vi "CTRE_Phoenix_CANcoder_ConfigAllSettings.vi"(6 "timeoutMs":i32=50, 7 "Force Write":bool, 8 "error in (no error)":errorcluster, 10 "CANcoder Configurables":T1={"Sensor Initialization Strategy"=enum."Boot To Zero", "Absolute Sensor Range"=enum."Unsigned [0 to 360)", "Velocity Measurement Period"=100, "Velocity Measurement Window"=64, "Magnet Offset (Degrees)"=0.0, "Sensor Direction"=FALSE, "Sensor Coefficient"=0.087890625, "Unit String"="deg", "Sensor Time Base"=enum."PerMinute"} {"Velocity Measurement Period" items=["Period_1ms"=1, "Period_2ms"=2, "Period_5ms"=5, "Period_10ms"=10, "Period_20ms"=20, "Period_25ms"=25, "Period_50ms"=50, "Period_100ms"=100]; "Sensor Coefficient" format="%#_9g"}, 11 "CTRE_CANcoder_DeviceRef":T6) -> (0 "error out":errorcluster, 3 "CTRE_CANcoder_DeviceRef":T6)   [LabVIEW 2019]
doc: "Configures all persistent settings of the CANcoder.\n\n<b>CANcoder Configurables</b> Cluster of configurable settings. Using a \"control\" on the calling VI's front panel will display documentation for each setting."
uses:
  <vilib>/Rock Robotics/WPI/ThirdParty/Phoenix-LabVIEW/CANCoder/Controls/CTRE_Phoenix_CANcoder_DeviceRef.ctl
  <vilib>/Rock Robotics/WPI/ThirdParty/Phoenix-LabVIEW/CANCoder/Controls/CTRE_Phoenix_CANcoder_Configurables.ctl
  <vilib>/Rock Robotics/WPI/ThirdParty/Phoenix-LabVIEW/CANCoder/Controls/CTRE_Phoenix_CANcoder_SensorInitializationStrategy.ctl
  <vilib>/Rock Robotics/WPI/ThirdParty/Phoenix-LabVIEW/CANCoder/Controls/CTRE_Phoenix_CANcoder_AbsoluteSensorRange.ctl
  <vilib>/Rock Robotics/WPI/ThirdParty/Phoenix-LabVIEW/Motor Controller/Controls/CTRE_Phoenix_MotorControl_VelocityMeasurementPeriod.ctl
  <vilib>/Rock Robotics/WPI/ThirdParty/Phoenix-LabVIEW/CANCoder/Controls/CTRE_Phoenix_CANcoder_SensorTimeBase.ctl
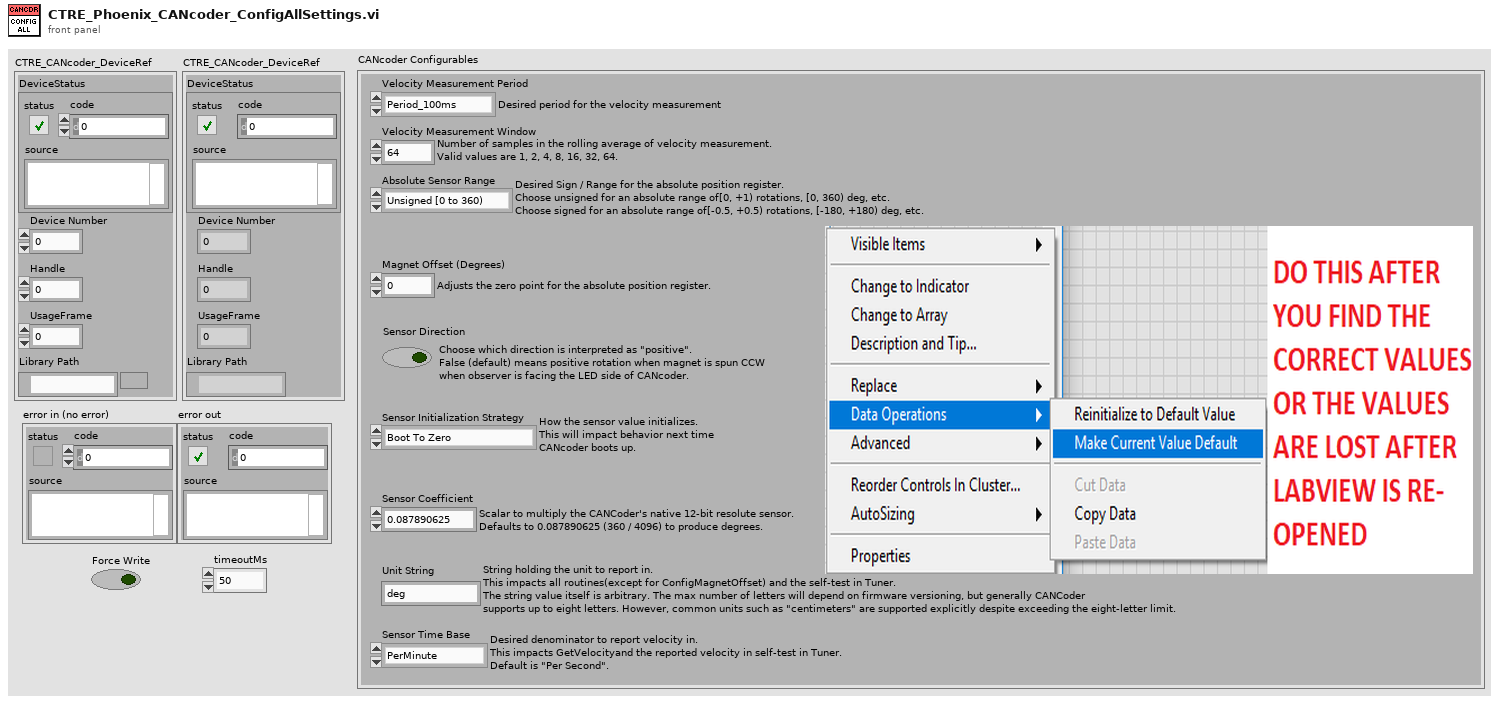
[diagram p1: front panel]
types:
  T1 = typedef "CTRE_Phoenix_CANcoder_Configurables.ctl" = cluster{"Sensor Initialization Strategy":T2, "Absolute Sensor Range":T3, "Velocity Measurement Period":T4, "Velocity Measurement Window":i32, "Magnet Offset (Degrees)":dbl, "Sensor Direction":bool, "Sensor Coefficient":dbl, "Unit String":string, "Sensor Time Base":T5}
  T2 = typedef "CTRE_Phoenix_CANcoder_SensorInitializationStrategy.ctl" = enum16{"Boot To Zero", "Boot To Absolute Position"}
  T3 = typedef "CTRE_Phoenix_CANcoder_AbsoluteSensorRange.ctl" = enum16{"Unsigned [0 to 360)", "Signed [-180 to +180)"}
  T4 = typedef "CTRE_Phoenix_MotorControl_VelocityMeasurementPeriod.ctl" = u16
  T5 = typedef "CTRE_Phoenix_CANcoder_SensorTimeBase.ctl" = enum16{"Per100Ms_Legacy", "PerSecond", "PerMinute"}
  T6 = typedef "CTRE_Phoenix_CANcoder_DeviceRef.ctl" = cluster{"DeviceStatus":errorcluster, "Device Number":u8, "Handle":u64, "UsageFrame":u32, "Library Path":path}
  T7 = cluster{"Sensor Initialization Strategy":bool, "Absolute Sensor Range":bool, "Velocity Measurement Period":bool, "Velocity Measurement Window":bool, "Magnet Offset (Degrees)":bool, "Sensor Direction":bool, "Sensor Coefficient":bool, "Unit String":bool, "Sensor Time Base":bool}
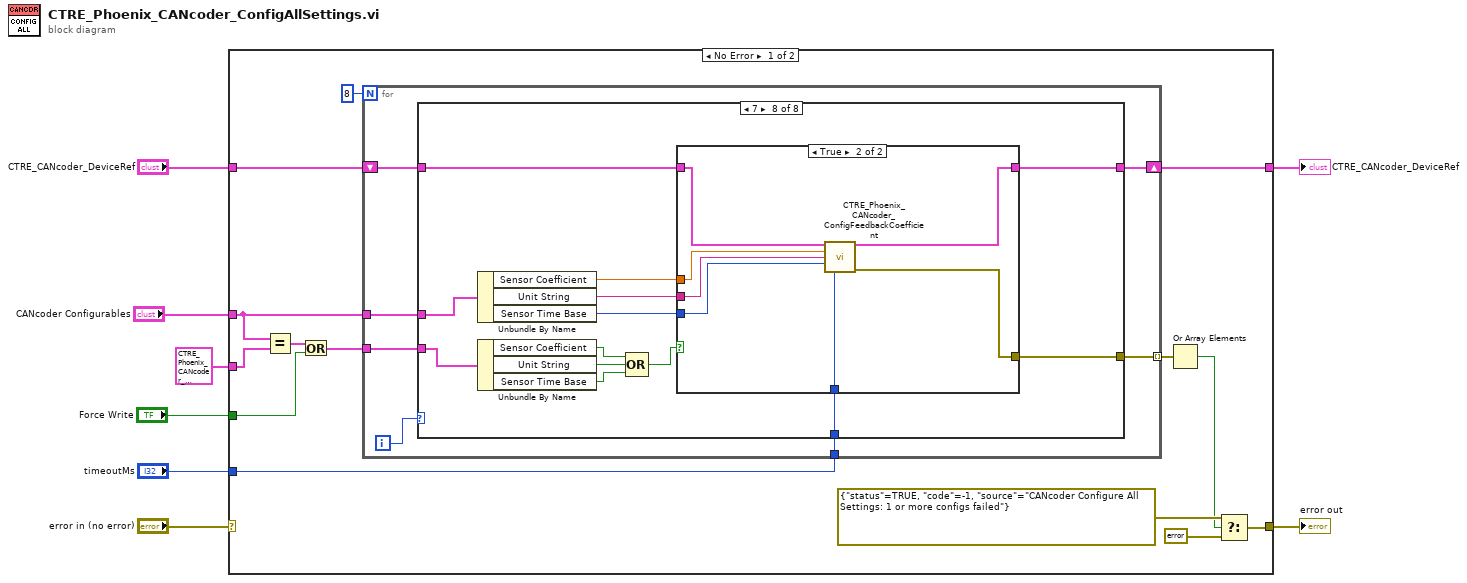
[diagram p0: block diagram]
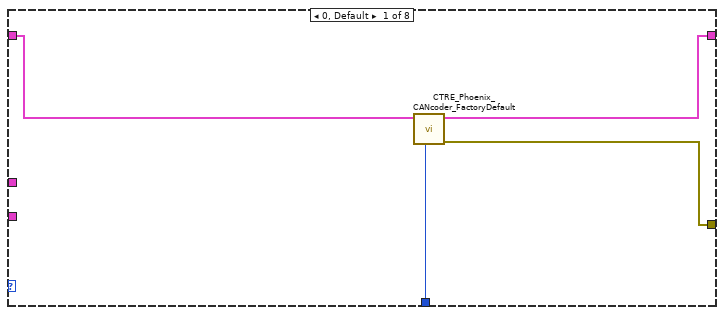
[diagram p2: hidden frame]
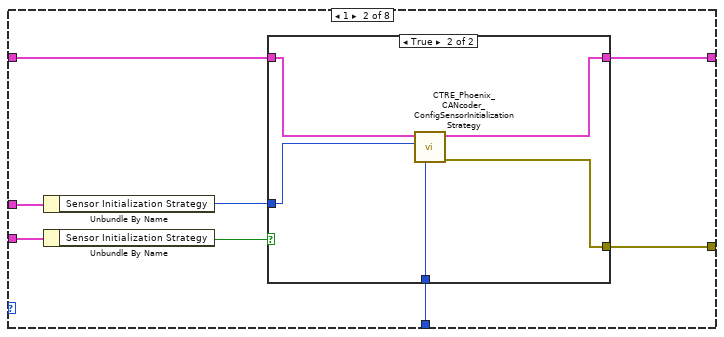
[diagram p3: hidden frame]
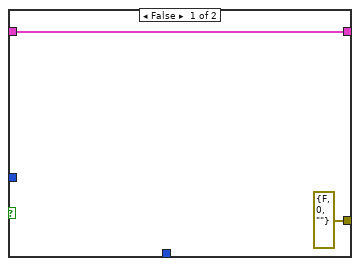
[diagram p4: hidden frame]
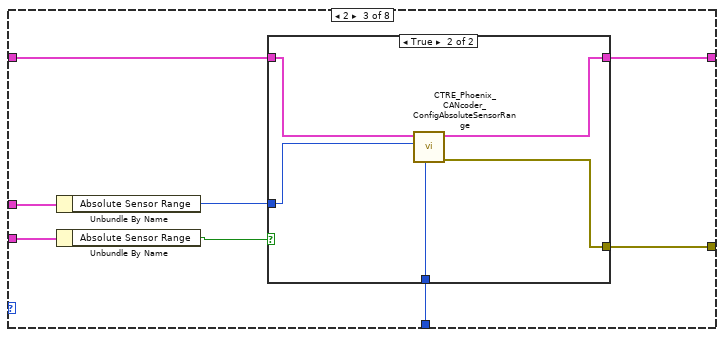
[diagram p5: hidden frame]
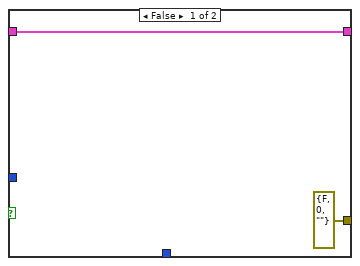
[diagram p6: hidden frame]
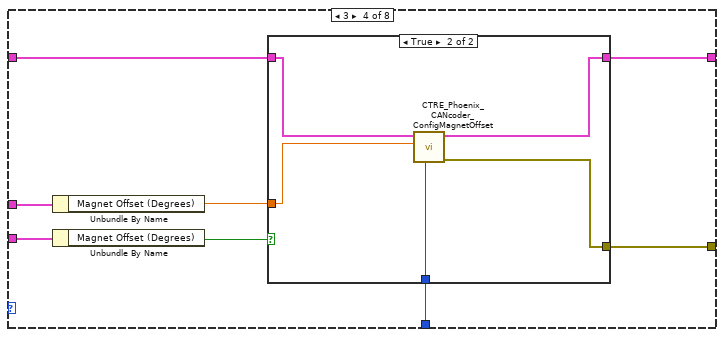
[diagram p7: hidden frame]
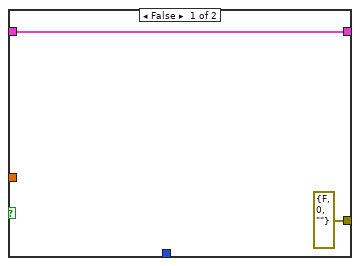
[diagram p8: hidden frame]
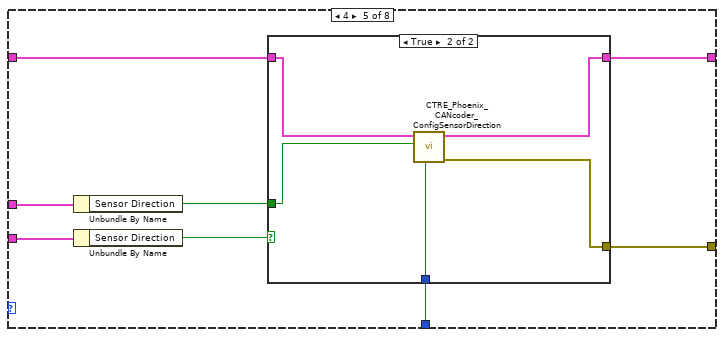
[diagram p9: hidden frame]
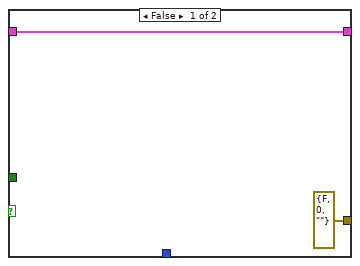
[diagram p10: hidden frame]
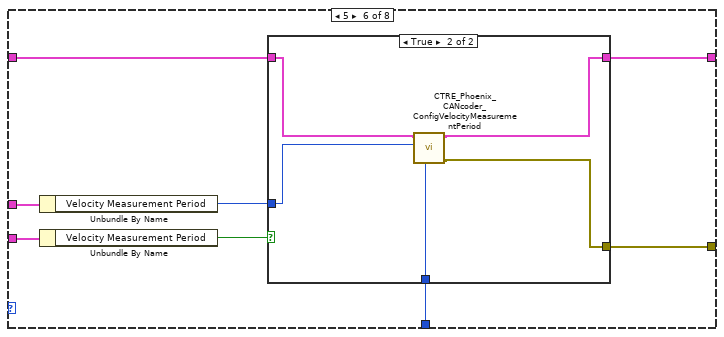
[diagram p11: hidden frame]
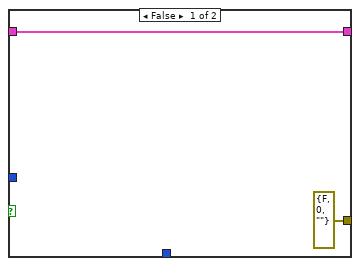
[diagram p12: hidden frame]
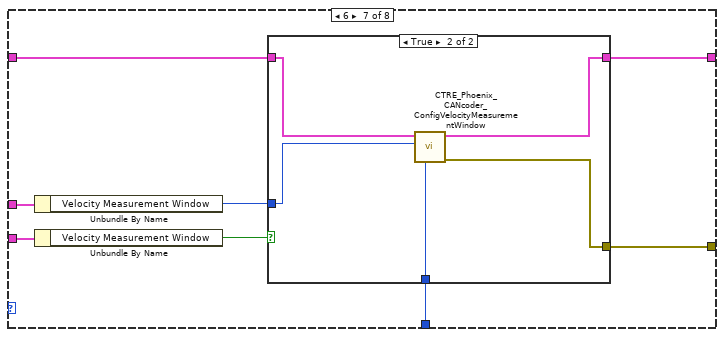
[diagram p13: hidden frame]
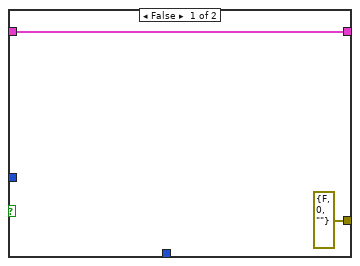
[diagram p14: hidden frame]
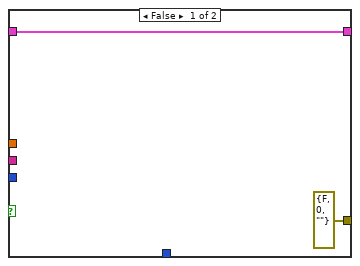
[diagram p15: hidden frame]
diagram:
  n1 = case shown="No Error" "error in (no error)" {
    selector: "error in (no error)" -> [_ w146]
    tunnel: "CTRE_CANcoder_DeviceRef" -> [w19 w147]
    tunnel: [w9 w147] -> w6
    tunnel: [w11 w146] -> w5
    tunnel: "timeoutMs" -> [w15 _]
    tunnel: "Force Write" -> [w20 _]
    tunnel: "CANcoder Configurables" -> [w16 _]
    tunnel: T1 {"Sensor Initialization Strategy"=enum."Boot To Zero", "Absolute Sensor Range"=enum."Unsigned [0 to 360)", "Velocity Measurement Period"=100, "Velocity Measurement Window"=64, "Magnet Offset (Degrees)"=0.0, "Sensor Direction"=FALSE, "Sensor Coefficient"=0.087890625, "Unit String"="deg", "Sensor Time Base"=enum."PerMinute"} ("CANcoder Configurables") -> [w22 _]
    frame No Error {
      n2 = Equal?(x=w16, y=w22) -> (x = y?=w21:T7)
      n3 = Or(x=w21, y=w20) -> (x .or. y?=w17:T7)
      n4 = for {
        N: 8 -> [_]
        shift-right: [w24] -> w9
        shift-left: w19 -> [w26]
        tunnel: w17 -> [w28]
        tunnel: w16 -> [w27]
        tunnel: w15 -> [w25]
        tunnel: [w23] -> w14 mode=indexing
        i -> [w29]
        n5 = case shown="7" w29 {
          tunnel: w28 -> [_ w40 w55 w70 w85 w100 w115 w135]
          tunnel: w27 -> [_ w41 w56 w71 w86 w101 w116 w136]
          tunnel: w26 -> [w32 w37 w52 w67 w82 w97 w112 w133]
          tunnel: w25 -> [w33 w35 w50 w65 w80 w95 w110 w131]
          tunnel: [w31 w36 w51 w66 w81 w96 w111 w132] -> w24
          tunnel: [w30 w34 w49 w64 w79 w94 w109 w130] -> w23
          frame 0, Default {
            n6 = call <vilib>:"CTRE_Phoenix_CANcoder_FactoryDefault.vi"("timeoutMs"=w33, "CTRE_CANcoder_DeviceRef"=w32) -> ("error out"=w30:errorcluster, "CTRE_CANcoder_DeviceRef"=w31:T6)  [unwired: 8 in]
          }
          frame 1 {
            n7 = Unbundle By Name(w41) -> ("Sensor Initialization Strategy"=w38:T2)
            n8 = Unbundle By Name(w40) -> ("Sensor Initialization Strategy"=w39:bool)
            n9 = case shown="True" w39 {
              tunnel: w38 -> [_ w45]
              tunnel: w37 -> [w43 w47]
              tunnel: [w43 w46] -> w36
              tunnel: w35 -> [_ w48]
              tunnel: [errorcluster {"status"=FALSE, "code"=0, "source"=""} ("error out") w44] -> w34
              frame False {
              }
              frame True {
                n10 = call <vilib>:"CTRE_Phoenix_CANcoder_ConfigSensorInitializationStrategy.vi"("timeoutMs"=w48, "Sensor Initialization Strategy"=w45, "CTRE_CANcoder_DeviceRef"=w47) -> ("error out"=w44:errorcluster, "CTRE_CANcoder_DeviceRef"=w46:T6)  [unwired: 7 in]
              }
            }
          }
          frame 2 {
            n11 = Unbundle By Name(w56) -> ("Absolute Sensor Range"=w53:T3)
            n12 = Unbundle By Name(w55) -> ("Absolute Sensor Range"=w54:bool)
            n13 = case shown="True" w54 {
              tunnel: w53 -> [_ w61]
              tunnel: w52 -> [w58 w63]
              tunnel: [w58 w62] -> w51
              tunnel: w50 -> [_ w60]
              tunnel: [errorcluster {"status"=FALSE, "code"=0, "source"=""} ("error out") w59] -> w49
              frame False {
              }
              frame True {
                n14 = call <vilib>:"CTRE_Phoenix_CANcoder_ConfigAbsoluteSensorRange.vi"("timeoutMs"=w60, "Absolute Sensor Range"=w61, "CTRE_CANcoder_DeviceRef"=w63) -> ("error out"=w59:errorcluster, "CTRE_CANcoder_DeviceRef"=w62:T6)  [unwired: 7 in]
              }
            }
          }
          frame 3 {
            n15 = Unbundle By Name(w71) -> ("Magnet Offset (Degrees)"=w68:dbl)
            n16 = Unbundle By Name(w70) -> ("Magnet Offset (Degrees)"=w69:bool)
            n17 = case shown="True" w69 {
              tunnel: w68 -> [_ w76]
              tunnel: w67 -> [w73 w78]
              tunnel: [w73 w77] -> w66
              tunnel: w65 -> [_ w74]
              tunnel: [errorcluster {"status"=FALSE, "code"=0, "source"=""} ("error out") w75] -> w64
              frame False {
              }
              frame True {
                n18 = call <vilib>:"CTRE_Phoenix_CANcoder_ConfigMagnetOffset.vi"("timeoutMs"=w74, "Magnet Offset (Degrees)"=w76, "CTRE_CANcoder_DeviceRef"=w78) -> ("error out"=w75:errorcluster, "CTRE_CANcoder_DeviceRef"=w77:T6)  [unwired: 7 in]
              }
            }
          }
          frame 4 {
            n19 = Unbundle By Name(w86) -> ("Sensor Direction"=w83:bool)
            n20 = Unbundle By Name(w85) -> ("Sensor Direction"=w84:bool)
            n21 = case shown="True" w84 {
              tunnel: w83 -> [_ w90]
              tunnel: w82 -> [w88 w92]
              tunnel: [w88 w91] -> w81
              tunnel: w80 -> [_ w93]
              tunnel: [errorcluster {"status"=FALSE, "code"=0, "source"=""} ("error out") w89] -> w79
              frame False {
              }
              frame True {
                n22 = call <vilib>:"CTRE_Phoenix_CANcoder_ConfigSensorDirection.vi"("timeoutMs"=w93, "Sensor Direction"=w90, "CTRE_CANcoder_DeviceRef"=w92) -> ("error out"=w89:errorcluster, "CTRE_CANcoder_DeviceRef"=w91:T6)  [unwired: 7 in]
              }
            }
          }
          frame 5 {
            n23 = Unbundle By Name(w101) -> ("Velocity Measurement Period"=w98:T4)
            n24 = Unbundle By Name(w100) -> ("Velocity Measurement Period"=w99:bool)
            n25 = case shown="True" w99 {
              tunnel: w98 -> [_ w104]
              tunnel: w97 -> [w103 w105]
              tunnel: [w103 w106] -> w96
              tunnel: w95 -> [_ w108]
              tunnel: [errorcluster {"status"=FALSE, "code"=0, "source"=""} ("error out") w107] -> w94
              frame False {
              }
              frame True {
                n26 = call <vilib>:"CTRE_Phoenix_CANcoder_ConfigVelocityMeasurementPeriod.vi"("timeoutMs"=w108, "Period"=w104, "CTRE_CANcoder_DeviceRef"=w105) -> ("error out"=w107:errorcluster, "CTRE_CANcoder_DeviceRef"=w106:T6)  [unwired: 7 in]
              }
            }
          }
          frame 6 {
            n27 = Unbundle By Name(w116) -> ("Velocity Measurement Window"=w113:i32)
            n28 = Unbundle By Name(w115) -> ("Velocity Measurement Window"=w114:bool)
            n29 = case shown="True" w114 {
              tunnel: w113 -> [_ w121]
              tunnel: w112 -> [w118 w123]
              tunnel: [w118 w122] -> w111
              tunnel: w110 -> [_ w119]
              tunnel: [errorcluster {"status"=FALSE, "code"=0, "source"=""} ("error out") w120] -> w109
              frame False {
              }
              frame True {
                n30 = call <vilib>:"CTRE_Phoenix_CANcoder_ConfigVelocityMeasurementWindow.vi"("timeoutMs"=w119, "windowSize"=w121, "CTRE_CANcoder_DeviceRef"=w123) -> ("error out"=w120:errorcluster, "CTRE_CANcoder_DeviceRef"=w122:T6)  [unwired: 7 in]
              }
            }
          }
          frame 7 {
            n31 = Unbundle By Name(w136) -> ("Sensor Coefficient"=w129:dbl, "Unit String"=w128:string, "Sensor Time Base"=w134:T5)
            n32 = Unbundle By Name(w135) -> ("Sensor Coefficient"=w127:bool, "Unit String"=w126:bool, "Sensor Time Base"=w125:bool)
            n33 = Compound Arithmetic op=OR(w127, w126, w125) -> (w124:bool)
            n34 = case shown="True" w124 {
              tunnel: w134 -> [_ w139]
              tunnel: w133 -> [w138 w145]
              tunnel: [w138 w144] -> w132
              tunnel: w131 -> [_ w143]
              tunnel: [errorcluster {"status"=FALSE, "code"=0, "source"=""} ("error out") w142] -> w130
              tunnel: w129 -> [_ w141]
              tunnel: w128 -> [_ w140]
              frame False {
              }
              frame True {
                n35 = call <vilib>:"CTRE_Phoenix_CANcoder_ConfigFeedbackCoefficient.vi"("CTRE_CANcoder_DeviceRef"=w145, "sensorCoefficient"=w141, "unitString"=w140, "timebase"=w139, "timeoutMs"=w143) -> ("CTRE_CANcoder_DeviceRef"=w144:T6, "error out"=w142:errorcluster)  [unwired: 9 in]
              }
            }
          }
        }
      }
      n36 = Or Array Elements(Boolean array=w14) -> (logical OR=w10:bool)
      n37 = Select(t=errorcluster {"status"=TRUE, "code"=-1, "source"="CANcoder Configure All Settings: 1 or more configs failed"} ("error out 2"), s=w10, f=errorcluster {"status"=FALSE, "code"=0, "source"=""} ("error out 2")) -> (s? t:f=w11:errorcluster)
    }
    frame Error {
    }
  }
  "CTRE_CANcoder_DeviceRef" <- w6
  "error out" <- w5
